vi "DER_SetPointQ_subTest.vi"(7 "Test Result in":T2=enum."Success", 8 "error in":errorcluster, 9 "DeviceID":T1, 10 "MicrogridID":u8, 11 "Message Enqueuer in":refnum<class "Message Enqueuer.lvclass">) -> (0 "error out":errorcluster, 1 "dup DeviceID":T1, 2 "dup MicrogridID":u8, 3 "Message Enqueuer out":refnum<class "Message Enqueuer.lvclass">, 5 "Test Result out":T2=enum."Success")   [LabVIEW 2018, in "IED Test Framework.lvlib" / "IED Test.lvclass"]
uses:
  IED Test.lvclass
  <vilib>/ActorFramework/Message Enqueuer/Message Enqueuer.lvclass
  Controls/Test Result.ctl
  <vilib>/ORNL/CSEISMIC DDS/CSEISMIC DDS Base/Data Types/Controls/DeviceID.ctl
  <vilib>/ORNL/CSEISMIC DDS/CSEISMIC DDS Base/Data Types/DER_SetPointQ.ctl
  <vilib>/ORNL/CSEISMIC DDS/CSEISMIC DDS Base/CSEISMIC DDS.lvclass/CSEISMIC DDS.ctl
  DER Actor/DER Messages/Write DER SetpointQ Msg/Write DER SetpointQ Msg.lvclass/Write DER SetpointQ Msg.ctl
  <vilib>/ActorFramework/Message Enqueuer/Message Enqueuer.lvclass/Message Enqueuer.ctl
  <vilib>/ORNL/CSEISMIC DDS/CSEISMIC DDS Base/Accessors/Write DDS Reference.vi
  <vilib>/ORNL/CSEISMIC DDS/CSEISMIC DDS Base/Accessors/Read DDS Reference.vi
  <vilib>/ActorFramework/Message Enqueuer/Enqueue.vi
  <vilib>/ORNL/CSEISMIC DDS/DDS Reader/DDS Reader.lvclass
  C:/Program Files (x86)/National Instruments/LabVIEW 2018/vi.lib/ORNL/CSEISMIC DDS/CSEISMIC DDS Base/CSEISMIC DDS.lvclass
  DER Actor/DER Messages/Write DER SetpointQ Msg/Write DER SetpointQ Msg.lvclass
  C:/Program Files (x86)/National Instruments/LabVIEW 2018/vi.lib/ActorFramework/Message/Message.lvclass
  <vilib>/ORNL/CSEISMIC DDS/CSEISMIC DDS Base/Error Handler.vi
  <vilib>/ActorFramework/Message Priority Queue/Priority Enqueue.vi
  <vilib>/ORNL/CSEISMIC DDS/CSEISMIC DDS Base/CSEISMIC DDS.lvclass
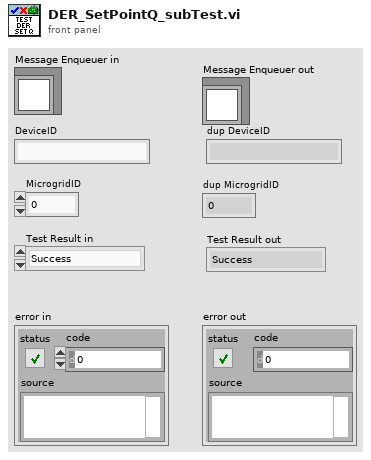
[diagram p1: front panel]
types:
  T1 = typedef "CSEISMIC DDS.lvlib/CSEISMIC DDS.lvclass/DeviceID.ctl" = string
  T2 = typedef "IED Test Framework.lvlib/IED Test.lvclass/Test Result.ctl" = enum16{"Invalid", "Success", "Failure", "Error", "Timeout"}
  T3 = typedef "CSEISMIC DDS.lvlib/CSEISMIC DDS.lvclass/DER_SetPointQ.ctl" = cluster{"DeviceID":T1, "ReactivePower (kVAR)":dbl[]}
  T4 = typedef "LVDDS_library.lvlib/DDS Sample Info.ctl" = cluster{"DDS_SampleStateKind":enum32{"DDS_INVALID_SAMPLE_STATE", "DDS_READ_SAMPLE_STATE", "DDS_NOT_READ_SAMPLE_STATE"}, "DDS_ViewStateKind":enum32{"DDS_INVALID_SAMPLE_STATE", "DDS_NEW_VIEW_STATE", "DDS_NOT_NEW_VIEW_STATE"}, "DDS_InstanceStateKind":enum32{"DDS_INVALID_STATE", "DDS_ALIVE_INSTANCE_STATE", "DDS_NOT_ALIVE_DISPOSED_INSTANCE_STATE", "", "DDS_NOT_ALIVE_NO_WRITERS_INSTANCE_STATE"}, "sec":i32, "nanosec":u32, "valid_data":bool}
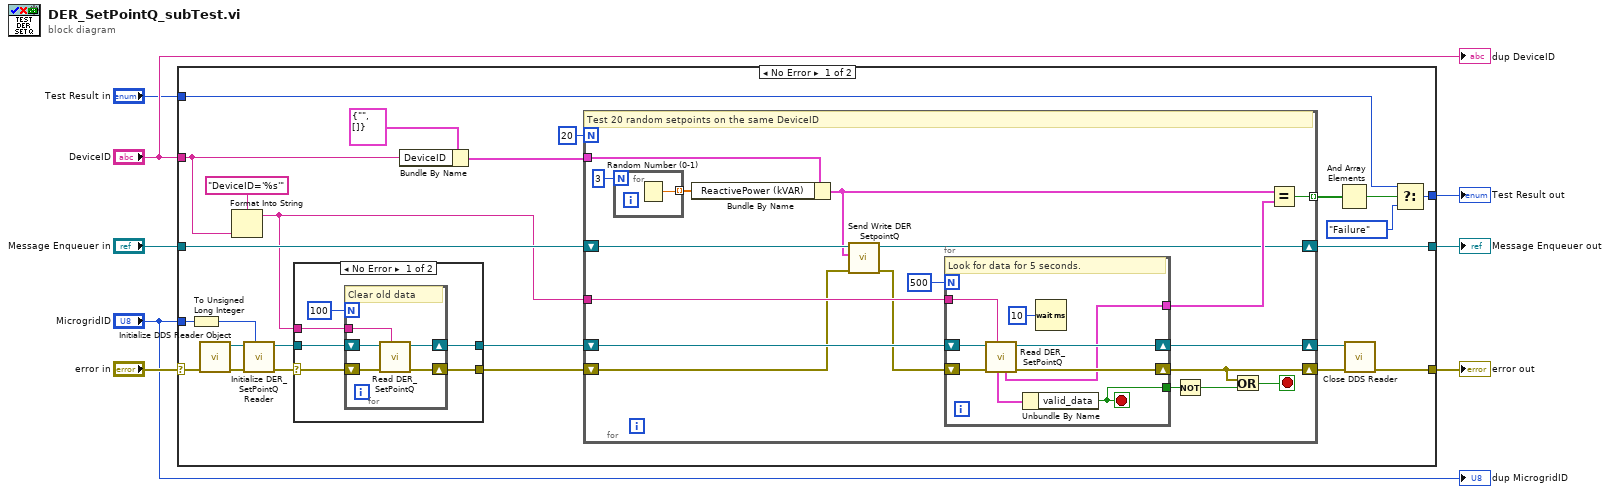
[diagram p0: block diagram]
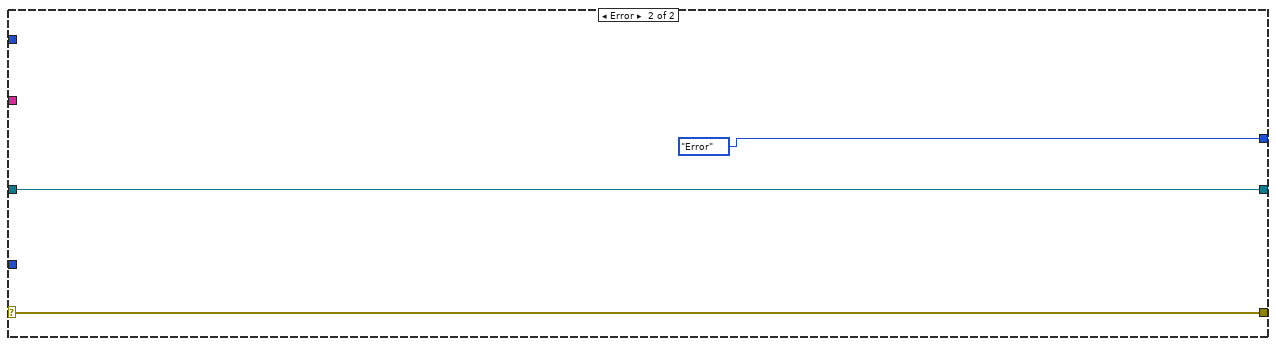
[diagram p3: hidden frame]
diagram:
  n1 = case shown="No Error" "error in" {
    selector: "error in" -> [w22 w77]
    tunnel: "Test Result in" -> [w28 _]
    tunnel: [w27 Test_Result."Error" ("f")] -> w6
    tunnel: "DeviceID" -> [w11 _]
    tunnel: "MicrogridID" -> [w18 _]
    tunnel: [w13 w77] -> w5
    tunnel: [w26 w76] -> w4
    tunnel: "Message Enqueuer in" -> [w25 w76]
    frame No Error {
      n2 = To Unsigned Long Integer(number=w18) -> (unsigned 32bit integer=w16:u32)
      n3 = call <vilib>:"Initialize DDS Reader Object.vi"("error in"=w22) -> ("error out"=w21:errorcluster, "DDS Reader out"=w19:refnum<class "DDS Reader.lvclass">)  [unwired: 9 in]
      n4 = Format Into String(format string="DeviceID='%s'", w11) -> (resulting string=w9:string)  [unwired: 2 in, 1 out]
      n5 = call <vilib>:"Initialize DER_SetPointQ Reader.vi"("MicrogridID"=w16, "error in"=w21, "DDS Reader in"=w19) -> ("error out"=w20:errorcluster, "DDS Reader out"=w17:refnum<class "DDS Reader.lvclass">)  [unwired: 7 in]
      n6 = case shown="No Error" w20 {
        selector: w20 -> [w67 w74]
        tunnel: [w66 w74] -> w30
        tunnel: w17 -> [w65 w73]
        tunnel: [w64 w73] -> w24
        tunnel: w9 -> [w62 _]
        frame No Error {
          n7 = for {
            N: 100 -> [_]
            shift-right: [w72] -> w66
            shift-left: w67 -> [w69]
            shift-right: [w70] -> w64
            shift-left: w65 -> [w71]
            tunnel: w62 -> [w68]
            # "Clear old data"
            n8 = call <vilib>:"Read DER_SetPointQ.vi"("Query condition"=w68, "error in"=w69, "DDS Reader in"=w71) -> ("error out"=w72:errorcluster, "DDS Reader out"=w70:refnum<class "DDS Reader.lvclass">)  [unwired: 5 in, 2 out]
          }
        }
        frame Error {
        }
      }
      n9 = Bundle By Name(cluster=T3 {"DeviceID"="", "ReactivePower (kVAR)"=[]} ("DER_SetPointQ"), "DeviceID"=w11) -> (w10:T3)
      n10 = for {
        N: 20 -> [_]
        tunnel: w10 -> [w42]
        tunnel: [w51] -> w33 mode=indexing
        shift-right: [w48] -> w15
        shift-left: w30 -> [w35]
        shift-right: [w49] -> w14
        shift-left: w24 -> [w50]
        shift-right: [w37] -> w26
        shift-left: w25 -> [w38]
        tunnel: w9 -> [w41]
        stop <- w46 stop-if-true
        # "Test 20 random setpoints on the same DeviceID"
        n11 = for {
          N: 3 -> [_]
          tunnel: [w52] -> w40 mode=indexing
          n12 = Random Number (0-1)() -> (number: 0 to 1=w52:dbl)
        }
        n13 = Bundle By Name(cluster=w42, "ReactivePower (kVAR)"=w40) -> (w34:T3)
        n14 = call "Send Write DER SetpointQ.vi"("error in (no error)"=w35, "DER_SetPointQ"=w34, "Message Enqueuer"=w38) -> ("error out"=w36:errorcluster, "Message Enqueuer out"=w37:refnum<class "Message Enqueuer.lvclass">)  [unwired: 7 in]
        n15 = for {
          N: 500 -> [_]
          tunnel: [w54] -> w45
          shift-right: [w57] -> w48
          shift-left: w36 -> [w60]
          shift-right: [w58] -> w49
          shift-left: w50 -> [w59]
          tunnel: [w55] -> w47
          tunnel: w41 -> [w53]
          stop <- w55 stop-if-true
          # "Look for data for 5 seconds."
          n16 = call <vilib>:"Read DER_SetPointQ.vi"("Query condition"=w53, "error in"=w60, "DDS Reader in"=w59) -> ("error out"=w57:errorcluster, "DDS Reader out"=w58:refnum<class "DDS Reader.lvclass">, "data"=w54:T3, "DDS Sample Info"=w56:T4)  [unwired: 5 in]
          n17 = Unbundle By Name(w56) -> ("valid_data"=w55:bool)
          n18 = Wait (ms)(milliseconds to wait=u32 10) -> ()  [unwired: 1 out]
        }
        n19 = Not(x=w47) -> (.not. x?=w43:bool)
        n20 = Or(x=w48, y=w43) -> (x .or. y?=w46:bool)
        n21 = Equal?(x=w34, y=w45) -> (x = y?=w51:bool)
      }
      n22 = And Array Elements(Boolean array=w33) -> (logical AND=w32:bool)
      n23 = call <vilib>:"Close DDS Reader.vi"("error in"=w15, "DDS Reader in"=w14) -> ("error out"=w13:errorcluster)  [unwired: 9 in]
      n24 = Select(t=w28, s=w32, f=Test_Result."Failure") -> (s? t:f=w27:T2)
    }
    frame Error {
    }
  }
  "Test Result out" <- w6
  "error out" <- w5
  "Message Enqueuer out" <- w4
  "dup DeviceID" <- "DeviceID"
  "dup MicrogridID" <- "MicrogridID"
